vi "Scaling_WF.vi"(8 "Axis_unit_1D":dbl[](array[numeric])=[0.0, 0.25, 0.5, 0.75, 1.0], 9 "FOV_Axis (µm)":dbl=100.0, 10 "Center Axis (µm)":dbl=50.0, 11 "Calib_Axis":dbl=0.1) -> (3 "Axis_volts":dbl[](array[numeric])=[0.0, 2.5, 5.0, 7.5, 10.0])   [LabVIEW 2026]
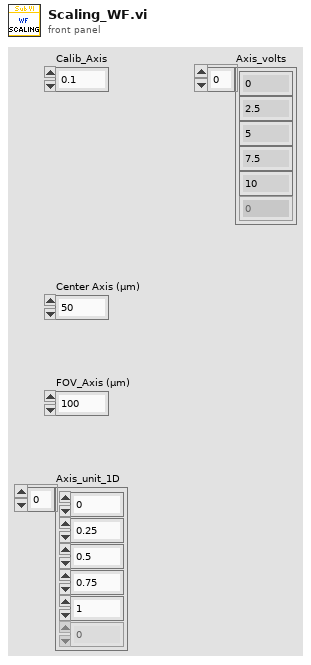
[diagram p1: front panel]
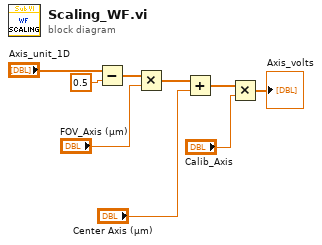
[diagram p0: block diagram]
diagram:
  n1 = Subtract(x="Axis_unit_1D", y=0.5) -> (x-y=w4:dbl[])
  n2 = Multiply(x=w4, y="FOV_Axis (µm)") -> (x*y=w6:dbl[])
  n3 = Add(x=w6, y="Center Axis (µm)") -> (x+y=w8:dbl[])
  n4 = Multiply(x=w8, y="Calib_Axis") -> (x*y=→"Axis_volts":dbl[])
